vi "Set Retardation.vi"(8 "error in (no error)":errorcluster, 10 "Retardation":dbl=1.0 min=0.0 max=1.0 step=0.001, 11 "VISA resource name":refnum<visa-resource-name>="COM1") -> (0 "error out":errorcluster, 2 "query output":string, 3 "VISA resource name out":refnum<visa-resource-name>)   [LabVIEW 2017]
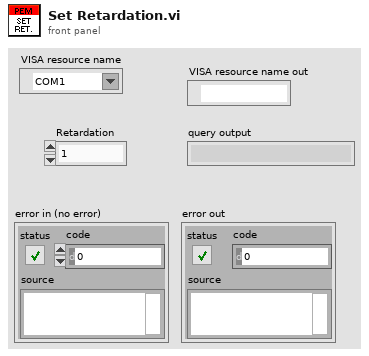
[diagram p1: front panel]
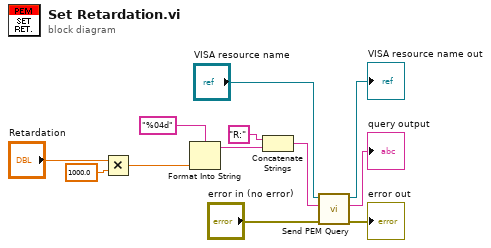
[diagram p0: block diagram]
diagram:
  n1 = Multiply(x="Retardation", y=1000.0) -> (x*y=w7:dbl)
  n2 = Format Into String(format string="%04d", w7) -> (resulting string=w10:string)  [unwired: 2 in, 1 out]
  n3 = Concatenate Strings("R:" ("write buffer"), w10) -> (w2:string)
  n4 = call "Send PEM Query.vi"("error in (no error)"="error in (no error)", "query string"=w2, "VISA resource name"="VISA resource name") -> ("error out"=→"error out":errorcluster, "query output"=→"query output":string, "VISA resource name out"=→"VISA resource name out":refnum<visa-resource-name>)  [unwired: 5 in, 1 out]
